vi "OperateClick.vi"(3 "XRef":refnum<vi>, 4 "Point":T1, 5 "State In":T3={"Input Type"=variant(dbl 0.0), "Selection"=0, "Element Names"=[], "Type Strings"=[], "Element Types"=[]}) -> (0 "Reply":string[](array[string]), 2 "State Out":T3={"Input Type"=variant(dbl 0.0), "Selection"=0, "Element Names"=[], "Type Strings"=[], "Element Types"=[]})   [LabVIEW 2015, in "Construct-Tagged-Union.xnode"]
doc: "This ability VI is called when a user operate clicks on your XNode. Point is the point of the click relative to the top-left corner of your XNode. If you wish to show a menu in response to a user's operate click, issue the reply \"ShowMenu\". It is an error to issue this reply if you have not implemented the BuildMenu and SelectMenu ability VIs.\n\nDefault behavior: None.\n\nThis ability provides UI and OS messages are handled.\n\nSee also: BuildMenu3, SelectMenu3"
uses:
  Construct-Tagged-Union.xnode
  State.ctl
  <vilib>/XNodeSupport/XNodePoint.ctl
  <vilib>/XNodeSupport/XNodeInt.ctl
  <vilib>/XNodeSupport/NI_XNodeSupport.lvlib
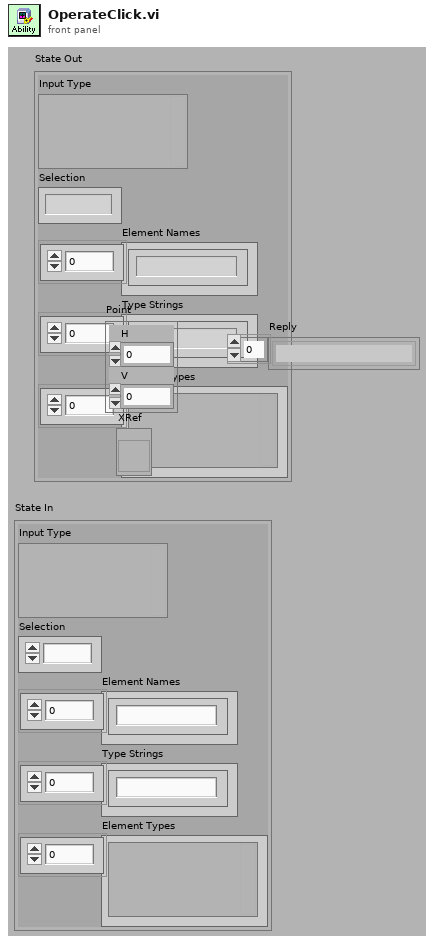
[diagram p1: front panel]
types:
  T1 = typedef "NI_XNodeSupport.lvlib/XNodePoint.ctl" = cluster{"H":T2, "V":T2}
  T2 = typedef "NI_XNodeSupport.lvlib/XNodeInt.ctl" = i32
  T3 = typedef "Construct-Tagged-Union.xnode/State.ctl" = cluster{"Input Type":variant, "Selection":i32, "Element Names":string[], "Type Strings":string[], "Element Types":variant[]}
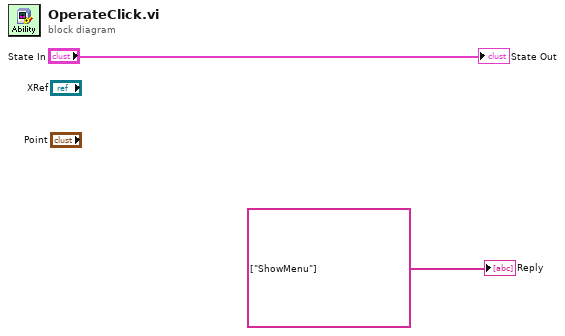
[diagram p0: block diagram]
diagram:
  "State Out" <- "State In"
  "Reply" <- string[] ["ShowMenu"] ("Reply")
